vi "CONV 2D Boolean Array to String.vi"(0 "2-D Boolean":bool[][](array[boolean]), 1 "Delimiters (,;)":string=",;", 5 "Boolean Type (0,1)":T1) -> (6 "String":string)   [LabVIEW 2017]
doc: "This routine converts a 2-D Boolean Array into a String list. There must be exactly 2 characters in the delimiters field. The first character is the Column Delimiter, and the second character is the Row Delimiter.\n\nExample:\n\n2-D Boolean Input:\n\nT T F\nF T F\n\nDelimiters:\n,;\n\nString Output:\n1,1,0;0,1,0"
uses:
  Type Defs/CONV Boolean Type Enum.ctl
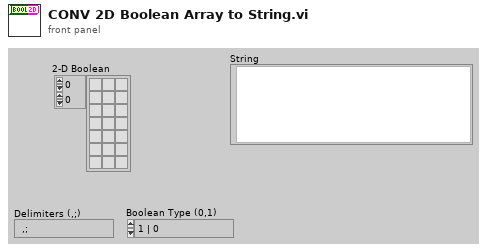
[diagram p1: front panel]
types:
  T1 = typedef "CONV Boolean Type Enum.ctl" = enum16{"1 | 0", "T | F", "True | False", "On | Off", "Yes | No"}
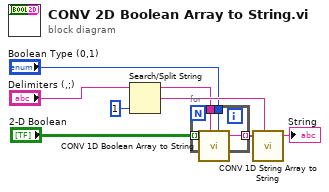
[diagram p0: block diagram]
diagram:
  n1 = Search/Split String(string="Delimiters (,;)", offset (0)=1) -> (substring before match=w2:string, match + rest of string=w3:string)  [unwired: 2 out]
  n2 = for {
    tunnel: "2-D Boolean" -> [w12] mode=indexing
    tunnel: [w11] -> w6 mode=indexing
    tunnel: w2 -> [w10]
    tunnel: "Boolean Type (0,1)" -> [w9]
    n3 = call "CONV 1D Boolean Array to String.vi"("1-D Boolean"=w12, "Delimiter (,)"=w10, "Boolean Type (1,0)"=w9) -> ("String"=w11:string)  [unwired: 6 out]
  }
  n4 = call "CONV 1D String Array to String.vi"("1-D String"=w6, "Delimiter (,)"=w3) -> ("String"=→"String":string)  [unwired: 7 out]
